vi "Send WebSocket Server-Service Enqueuer.vi"(5 "Receive Service/Server Enqueuer Handler":refnum<class "WebSocket Server-Service Enqueuer Msg.lvclass">, 6 "Service Name":string, 7 "Message Priority (Normal)":T1=enum."Normal", 8 "error in (no error)":errorcluster, 9 "Error":errorcluster, 10 "WebSocket Server/Service Enqueuer":refnum<class "Message Enqueuer.lvclass">, 11 "Message Enqueuer":refnum<class "Message Enqueuer.lvclass">) -> (0 "error out":errorcluster, 3 "Message Enqueuer out":refnum<class "Message Enqueuer.lvclass">)   [LabVIEW 2016, in "WebSocket Actors.lvlib" / "WebSocket Server-Service Enqueuer Msg.lvclass"]
doc: "This VI sends the message to an actor."
uses:
  WebSocket Server-Service Enqueuer Msg.lvclass
  <vilib>/ActorFramework/Message Enqueuer/Message Enqueuer.lvclass
  <vilib>/ActorFramework/Message Enqueuer/Message Priority.ctl
  C:/Program Files (x86)/National Instruments/LabVIEW 2016/vi.lib/ActorFramework/Message/Message.lvclass
  WebSocket Server-Service Enqueuer Msg.lvclass/WebSocket Server-Service Enqueuer Msg.ctl
  <vilib>/ActorFramework/Message Enqueuer/Message Enqueuer.lvclass/Message Enqueuer.ctl
  <vilib>/ActorFramework/Message Priority Queue/Priority Enqueue.vi
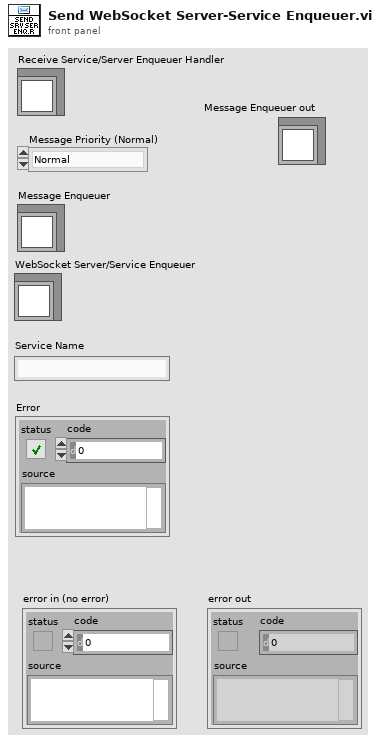
[diagram p1: front panel]
types:
  T1 = typedef "Actor Framework.lvlib/Message Enqueuer.lvclass/Message Priority.ctl" = enum16{"Low", "Normal", "High"}
  T2 = cluster{"Server/Service Enqueuer":refnum<class "Message Enqueuer.lvclass">, "Server/Service Name":string, "Error ":errorcluster}
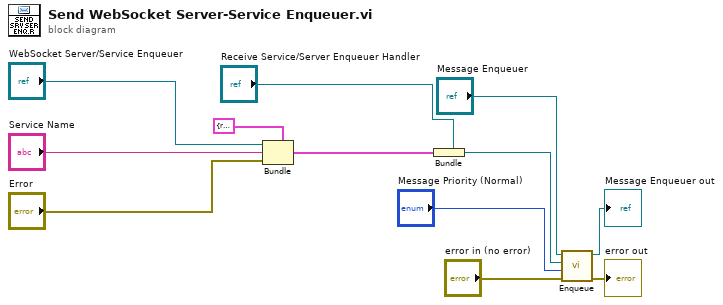
[diagram p0: block diagram]
diagram:
  n1 = Bundle(cluster=T2 {"Server/Service Enqueuer"=refnum, "Server/Service Name"="", "Error "={"status"=FALSE, "code"=0, "source"=""}} ("Server/Manager Response"), "Server/Service Enqueuer"="WebSocket Server/Service Enqueuer", "Server/Service Name"="Service Name", "Error"="Error") -> (w4:T2)
  n2 = Bundle(cluster="Receive Service/Server Enqueuer Handler", w4) -> (w8:refnum<class "WebSocket Server-Service Enqueuer Msg.lvclass">)
  n3 = call <vilib>:"Enqueue.vi"("error in (no error)"="error in (no error)", "Message Priority (Normal)"="Message Priority (Normal)", "Message"=w8, "Message Enqueuer in"="Message Enqueuer") -> ("error out"=→"error out":errorcluster, "Message Enqueuer out"=→"Message Enqueuer out":refnum<class "Message Enqueuer.lvclass">)  [unwired: 6 in]
